vi "sound_output_demo.vi"   [LabVIEW 2014]
uses:
  <vilib>/sound2/lvsound2.llb/Sound Output Write (DBL Single).vi
types:
  T1 = typedef "Sound Output Task ID.ctl" = u32
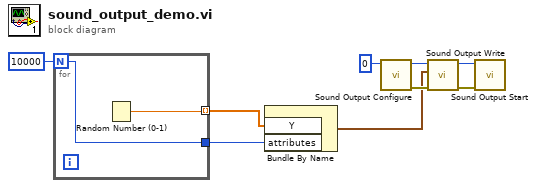
[diagram p0: block diagram]
diagram:
  n1 = for {
    N: 10000 -> [w11]
    tunnel: [w11] -> w8
    tunnel: [w10] -> w7 mode=indexing
    n2 = Random Number (0-1)() -> (number: 0 to 1=w10:dbl)
  }
  n3 = Bundle By Name("Y"=w7, "attributes"=w8) -> (w1:waveform(dbl))  [unwired: 1 in]
  n4 = call <vilib>:"Sound Output Configure.vi"("device ID"=u32 0) -> ("error out"=w5:errorcluster, "task ID"=w4:T1)  [unwired: 9 in]
  n5 = call-poly <vilib>:"Sound Output Write.vi"("error in (no error)"=w5, "data"=w1, "task ID"=w4) -> ("error out"=w3:errorcluster, "task ID out"=w2:T1)  [unwired: 7 in]
  n6 = call <vilib>:"Sound Output Start.vi"("error in (no error)"=w3, "task ID"=w2) -> ()  [unwired: 8 in, 2 out]
